vi "copy database to platform.vi"() -> ()   [LabVIEW 2016]
panel:
  out "error out":errorcluster
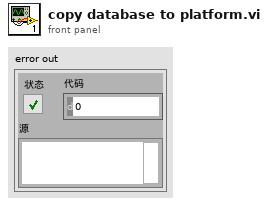
[diagram p1: front panel]
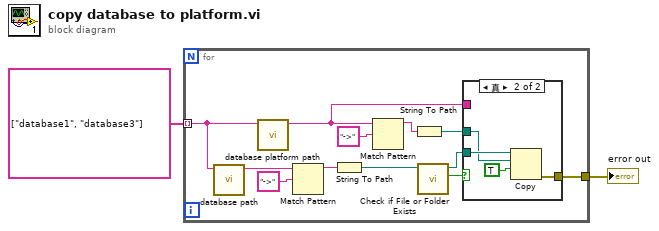
[diagram p0: block diagram]
diagram:
  n1 = for {
    tunnel: string[] ["database1", "database3"] -> [w11] mode=indexing
    tunnel: [w14] -> w1
    n2 = call "database path.vi"("database"=w11) -> ("Path out"=w7:string)  [unwired: 9 in, 1 out]
    n3 = call "database platform path.vi"("database"=w11) -> ("Path out"=w10:string)  [unwired: 10 in]
    n4 = Match Pattern(string=w7, regular expression="->") -> (before substring=w6:string)  [unwired: 1 in, 3 out]
    n5 = String To Path(string=w6) -> (path=w4:path)
    n6 = Match Pattern(string=w10, regular expression="->") -> (before substring=w5:string)  [unwired: 1 in, 3 out]
    n7 = String To Path(string=w5) -> (path=w3:path)
    n8 = call <vilib>:"Check if File or Folder Exists.vi"("path"=w4) -> ("file or folder exists?"=w13:bool, "dup path"=w12:path)  [unwired: 8 in, 1 out]
    n9 = case shown="真" w13 {
      tunnel: w10 -> [_ _]
      tunnel: [_ w17] -> w14
      tunnel: w12 -> [_ w16]
      tunnel: w3 -> [_ w15]
      frame False {
      }
      frame True {
        n10 = Copy(9:TRUE ("覆盖(F)"), 10:w15, 11:w16) -> (0:w17:errorcluster)  [unwired: 2 in, 2 out]
      }
    }
  }
  "error out" <- w1
